vi "Read Measure Binary.vi"(0 "VISA resource name":refnum<visa-resource-name>, 5 "Header (F: OFF)":bool, 11 "error in (no error)":errorcluster) -> (2 "Phase info.":u16[](array[ring]) items=["Lag", "Lead", "Cannot be detected"], 3 "Data status":u16[](array[ring]) items=["Normal", "Over range", "Voltage peak over", "Current peak over", "Power factor error", "Phase angle error", "Frequency error (Lo)", "Frequency error (Hi)", "Computation overflow", "PLL error", "No data"], 4 "VISA resource name out":refnum<visa-resource-name>, 6 "Read Data":string, 8 "Measure Value":sgl[](array[numeric]) format="%^.3e", 13 "Decimal Point":u16[](array[ring]) items=["_ _ _ _ _.", "_ _ _ _._", "_ _ _._ _", "_ _._ _ _", "_._ _ _ _", "._ _ _ _ _"], 14 "Prefix uint":u16[](array[ring]) items=["None", "m", "k", "M"], 15 "error out":errorcluster)   [LabVIEW 2016, in "Yokogawa WT200 Series.lvlib"]
doc: "This VI reads the Measure Binary Value from the WT210/WT230."
uses:
  Yokogawa WT200 Series.lvlib
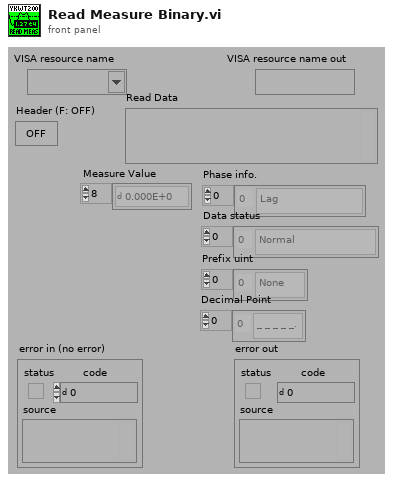
[diagram p1: front panel]
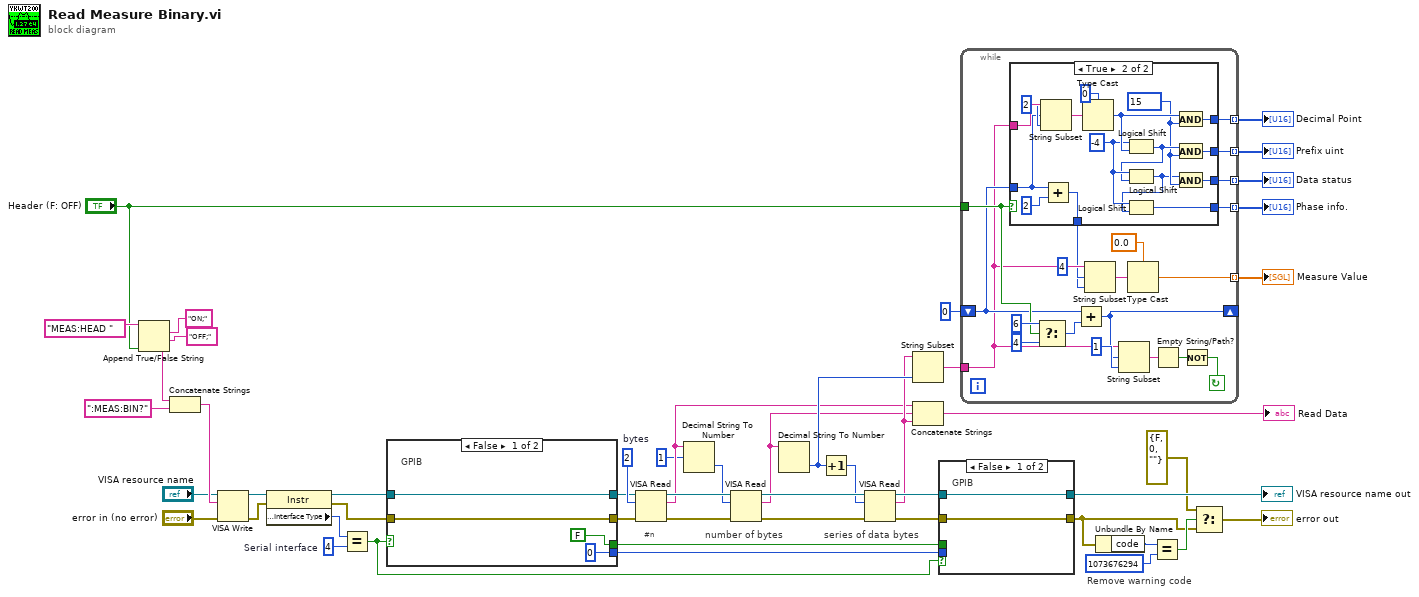
[diagram p0: block diagram]
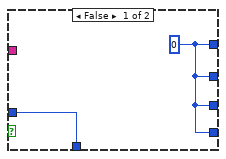
[diagram p2: hidden frame]
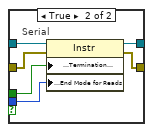
[diagram p3: hidden frame]
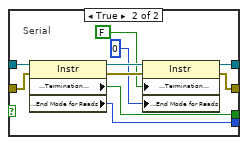
[diagram p4: hidden frame]
diagram:
  w33 = u16 4  # Serial interface
  w47 = u32 2  # bytes
  # "#n"
  # "series of data bytes"
  # "number of bytes"
  # "Remove warning code"
  n1 = Append True/False String(1:"Header (F: OFF)", 2:"OFF;", 3:"ON;", 4:"MEAS:HEAD ") -> (0:w42:string)
  n2 = Concatenate Strings(w42, ":MEAS:BIN?") -> (w44:string)
  n3 = VISA Write(VISA resource name="VISA resource name", write buffer=w44, error in (no error)="error in (no error)") -> (VISA resource name out=w23:refnum<visa-resource-name>, error out=w24:errorcluster)  [unwired: 1 out]
  n4 = property class="Instr"(reference=w23, error in=w24) -> (reference out=w32:refnum<visa-resource-name>, error out=w31:errorcluster, "Interface Information:Interface Type"=w34:u16)
  n5 = Equal?(x=w34, y=w33) -> (x = y?=w30:bool)
  n6 = case shown="False" w30 {
    tunnel: [FALSE w62] -> w29
    tunnel: [w53 w60] -> w27
    tunnel: [w52 w59] -> w26
    tunnel: w32 -> [w53 w58]
    tunnel: w31 -> [w52 w57]
    tunnel: [u16 0 ("ASRL End In") w54] -> w7
    frame False {
      # "GPIB"
    }
    frame True {
      # "Serial"
      n7 = property class="Instr"(reference=w58, error in=w57) -> (reference out=w61:refnum<visa-resource-name>, error out=w63:errorcluster, "Message Based Settings:Termination Character Enable"=w62:bool, "Serial Settings:End Mode for Reads"=w54:u16)
      n8 = property class="Instr"(reference=w61, error in=w63, "Message Based Settings:Termination Character Enable"=FALSE ("TermChar"), "Serial Settings:End Mode for Reads"=u16 0 ("ASRL End In")) -> (reference out=w60:refnum<visa-resource-name>, error out=w59:errorcluster)
    }
  }
  n9 = VISA Read(VISA resource name=w27, byte count=w47, error in (no error)=w26) -> (VISA resource name out=w21:refnum<visa-resource-name>, read buffer=w11:string, error out=w18:errorcluster)  [unwired: 1 out]
  n10 = Decimal String To Number(string=w11, offset=1) -> (number=w15:i32)  [unwired: 1 in, 1 out]
  n11 = VISA Read(VISA resource name=w21, byte count=w15, error in (no error)=w18) -> (VISA resource name out=w20:refnum<visa-resource-name>, read buffer=w10:string, error out=w17:errorcluster)  [unwired: 1 out]
  n12 = Decimal String To Number(string=w10) -> (number=w14:i32)  [unwired: 2 in, 1 out]
  n13 = Increment(x=w14) -> (x+1=w8:i32)
  n14 = VISA Read(VISA resource name=w20, byte count=w8, error in (no error)=w17) -> (VISA resource name out=w19:refnum<visa-resource-name>, read buffer=w13:string, error out=w16:errorcluster)  [unwired: 1 out]
  n15 = String Subset(string=w13, length (rest)=w14) -> (substring=w40:string)  [unwired: 1 in]
  n16 = Concatenate Strings(w11, w10, w13) -> (→"Read Data":string)
  n17 = case shown="False" w30 {
    tunnel: w19 -> [w65 w71]
    tunnel: w16 -> [w64 w70]
    tunnel: [w65 w68] -> w28
    tunnel: w29 -> [_ w69]
    tunnel: [w64 w66] -> w3
    tunnel: w7 -> [_ w67]
    frame False {
      # "GPIB"
    }
    frame True {
      # "Serial"
      n18 = property class="Instr"(reference=w71, error in=w70, "Message Based Settings:Termination Character Enable"=w69, "Serial Settings:End Mode for Reads"=w67) -> (reference out=w68:refnum<visa-resource-name>, error out=w66:errorcluster)
    }
  }
  "VISA resource name out" <- w28
  n19 = while {
    tunnel: [w72] -> w35 mode=indexing
    tunnel: [w73] -> w36 mode=indexing
    tunnel: [w74] -> w37 mode=indexing
    tunnel: [w75] -> w38 mode=indexing
    tunnel: "Header (F: OFF)" -> [w83]
    tunnel: [w76] -> w48 mode=indexing
    shift-left: u32 0 -> [w82]
    shift-right: [w87] -> _
    tunnel: w40 -> [w81]
    stop <- w88 continue-if-true
    n20 = case shown="True" w83 {
      tunnel: w81 -> [_ w109]
      tunnel: w82 -> [w93 w100]
      tunnel: [w93 w98] -> w80
      tunnel: [w92 w97] -> w75
      tunnel: [w92 w96] -> w74
      tunnel: [w92 w95] -> w73
      tunnel: [w92 w94] -> w72
      frame False {
        w92 = u16 0
      }
      frame True {
        w104 = i16 -4
        w102 = u16 15
        n21 = String Subset(string=w109, offset (0)=w100, length (rest)=2) -> (substring=w107:string)
        n22 = Add(x=w100, y=u32 2) -> (x+y=w98:u32)
        n23 = Type Cast(type=u16 0, x=w107) -> (*(type *) &x=w105:u16)
        n24 = Logical Shift(y=w104, x=w105) -> (x << y=w103:u16)
        n25 = Logical Shift(y=w104, x=w103) -> (x << y=w101:u16)
        n26 = Logical Shift(y=w104, x=w101) -> (x << y=w94:u16)
        n27 = And(x=w105, y=w102) -> (x .and. y?=w97:u16)
        n28 = And(x=w103, y=w102) -> (x .and. y?=w96:u16)
        n29 = And(x=w101, y=w102) -> (x .and. y?=w95:u16)
      }
    }
    n30 = Select(t=u32 6, s=w83, f=u32 4) -> (s? t:f=w86:u32)
    n31 = Add(x=w82, y=w86) -> (x+y=w87:u32)
    n32 = String Subset(string=w81, offset (0)=w80, length (rest)=4) -> (substring=w78:string)
    n33 = String Subset(string=w81, offset (0)=w87, length (rest)=1) -> (substring=w90:string)
    n34 = Type Cast(type=sgl 0.0, x=w78) -> (*(type *) &x=w76:sgl)
    n35 = Empty String/Path?(string/path=w90) -> (empty?=w89:bool)
    n36 = Not(x=w89) -> (.not. x?=w88:bool)
  }
  "Measure Value" <- w48
  "Phase info." <- w35
  "Data status" <- w36
  "Prefix uint" <- w37
  "Decimal Point" <- w38
  n37 = Unbundle By Name(w3) -> ("code"=w6:i32)
  n38 = Equal?(x=w6, y=1073676294 ("x")) -> (x = y?=w4:bool)
  n39 = Select(t=errorcluster {"status"=FALSE, "code"=0, "source"=""}, s=w4, f=w3) -> (s? t:f=→"error out":errorcluster)
